vi "Reentrancy Settings for Hierarchy.vi"(8 "error in":errorcluster, 11 "Scratch VI":refnum<vi>) -> (0 "error out":errorcluster, 3 "Reentrancy Settings for VI Hierarchy":T1[](array[typedef]))   [LabVIEW 2009]
uses:
  VI Reentrancy Setting.ctl
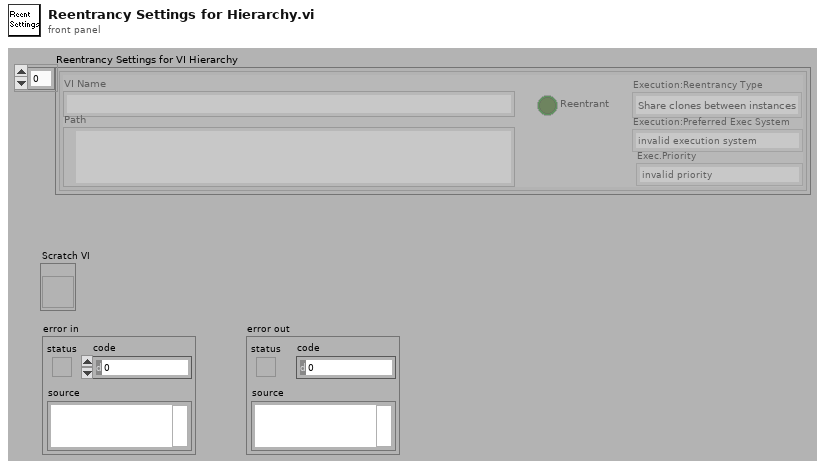
[diagram p1: front panel]
types:
  T1 = typedef "VI Reentrancy Setting.ctl" = cluster{"VI Name":string, "Path":path, "Reentrant":bool, "Execution:Reentrancy Type":enum16{"Share clones between instances", "Preallocate clone for each instance"}, "Execution:Preferred Exec System":enum32{"invalid execution system", "user interface", "standard", "instrument i/o", "data acquisition", "other 1", "other 2", "same as caller"}, "Exec.Priority":enum32{"invalid priority", "background priority", "normal priority", "above normal priority", "high priority", "time critical priority", "subroutine"}}
  T2 = enum8{"Only include commented out diagrams if diagram already loaded", "Never include commented out diagrams", "Always include commented out diagrams"}
  T3 = enum8{"No dynamic dispatch VIs", "Include nearest implementation", "Include all overrides"}
  T4 = enum8{"Include the clone VI", "Include the original reentrant VI instead of the clone VI", "Include both the original reentrant VI and the clone VI"}
  T5 = enum16{"Share clones between instances", "Preallocate clone for each instance"}
  T6 = enum32{"invalid execution system", "user interface", "standard", "instrument i/o", "data acquisition", "other 1", "other 2", "same as caller"}
  T7 = enum32{"invalid priority", "background priority", "normal priority", "above normal priority", "high priority", "time critical priority", "subroutine"}
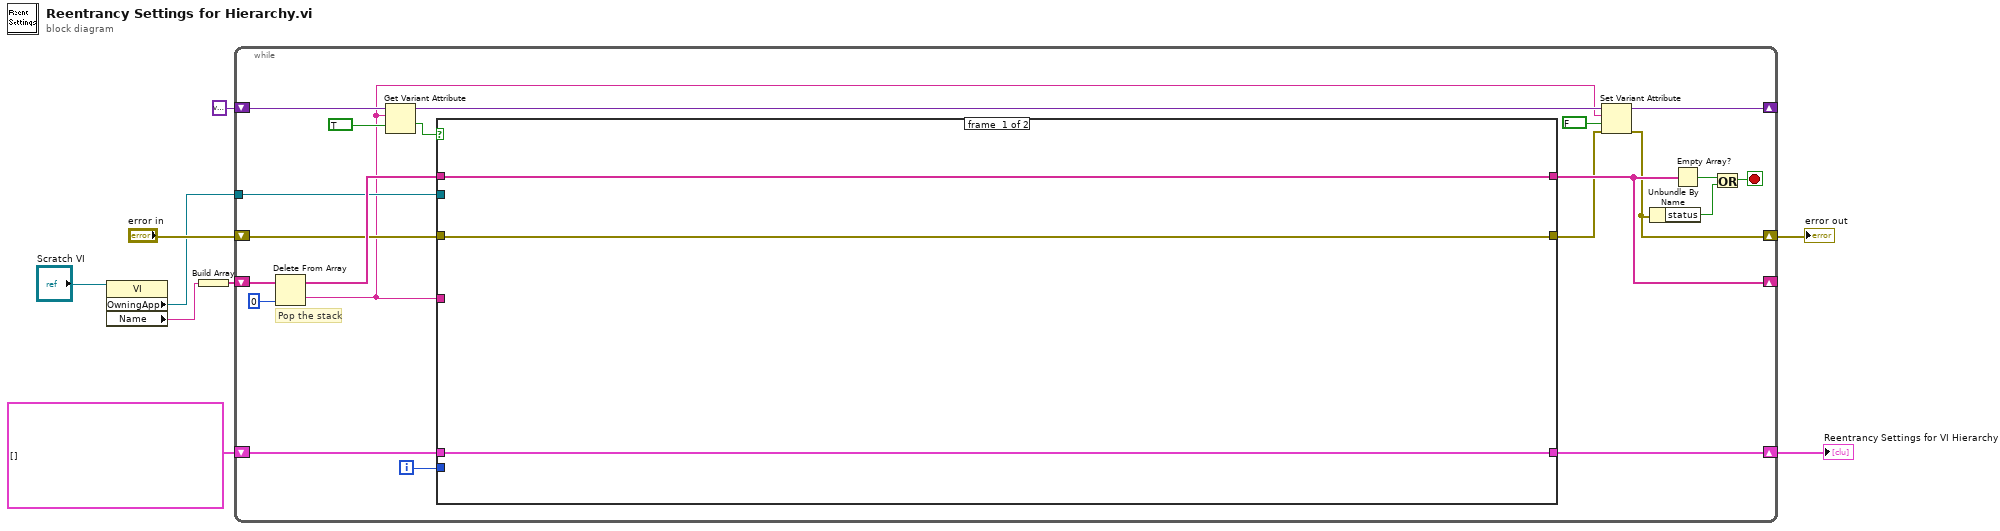
[diagram p0: block diagram]
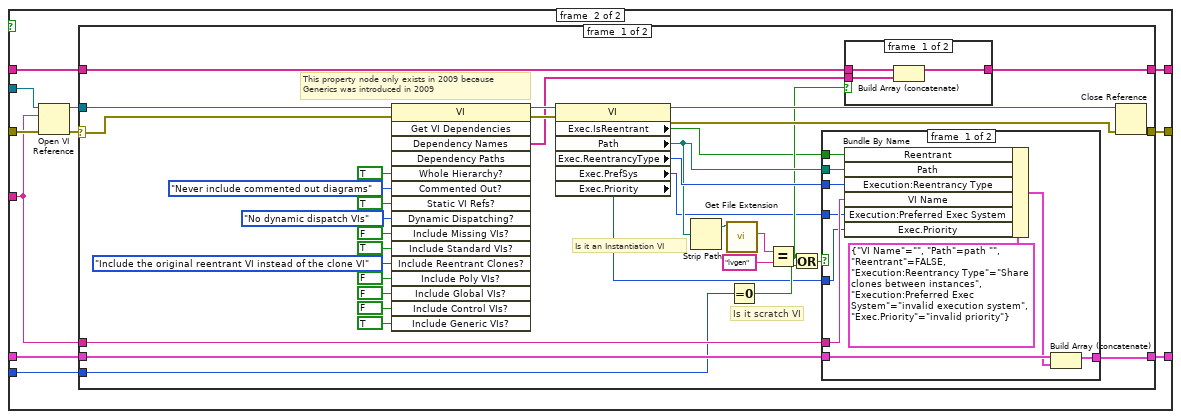
[diagram p2: hidden frame]
diagram:
  n1 = property class="VI"(reference="Scratch VI") -> ("OwningApp"=w2:refnum<vi>, "Name"=w3:string)  [unwired: 1 in, 2 out]
  n2 = Build Array(w3) -> (w4:string[])
  n3 = while {
    shift-right: [w28] -> _
    shift-left: w4 -> [w26]
    shift-right: [w23] -> w9
    shift-left: T1[] [] ("Array") -> [w30]
    shift-right: [w12] -> w8
    shift-left: "error in" -> [w17]
    tunnel: w2 -> [w24]
    shift-right: [w14] -> _
    shift-left: variant -> [w22]
    i -> [w15]
    stop <- w16 stop-if-true
    # "Pop the stack"
    n4 = Delete From Array(array=w26, index=0) -> (deleted portion=w11:string, array with subset deleted=w25:string[])  [unwired: 1 in]
    n5 = Get Variant Attribute(Variant=w22, name=w11, default value (empty Variant)=TRUE) -> (duplicate Variant=w21:variant, value=w19:bool)  [unwired: 1 in, 2 out]
    n6 = case shown="True" w19 {
      tunnel: w30 -> [w31 w36]
      tunnel: [w32 w43] -> w28
      tunnel: [w33 w42] -> w13
      tunnel: w17 -> [w33 w40]
      tunnel: w25 -> [w32 w39]
      tunnel: w24 -> [_ w38]
      tunnel: w11 -> [_ w37]
      tunnel: [w31 w35] -> w23
      tunnel: w15 -> [_ w34]
      frame #0 {
      }
      frame #1 {
        n7 = Open VI Reference(application reference (local)=w38, vi path=w37, error in (no error)=w40) -> (vi reference=w44:refnum<vi>, error out=w41:errorcluster)  [unwired: 3 in]
        n8 = case shown="No Error" w41 {
          selector: w41 -> [w60 w96]
          tunnel: w44 -> [w61 _]
          tunnel: w39 -> [w80 w98]
          tunnel: [w79 w98] -> w43
          tunnel: [w78 w96] -> w42
          tunnel: w37 -> [w77 _]
          tunnel: w36 -> [w76 w97]
          tunnel: [w75 w97] -> w35
          tunnel: w34 -> [w55 _]
          frame #0 {
            # "Is it an Instantiation VI"
            # "Is it scratch VI"
            # "This property node only exists in 2009 because\nGenerics was introduced in 2009"
            n9 = invoke class="VI" method="Get VI Dependencies"(reference=w61, error in=w60, "Whole Hierarchy?"=TRUE, "Commented Out?"=T2."Never include commented out diagrams" ("Commented Out Diagrams?"), "Static VI Refs?"=TRUE, "Dynamic Dispatching?"=T3."No dynamic dispatch VIs", "Include Missing VIs?"=FALSE ("Include Missing Items?"), "Include Standard VIs?"=TRUE, "Include Reentrant Clones?"=T4."Include the original reentrant VI instead of the clone VI", "Include Poly VIs?"=FALSE, "Include Global VIs?"=FALSE, "Include Control VIs?"=FALSE, "Include Generic VIs?"=TRUE) -> (reference out=w58:refnum<vi>, error out=w59:errorcluster, "Dependency Names"=w57:string[])  [unwired: 3 in, 13 out]
            n10 = property class="VI"(reference=w58, error in=w59) -> (reference out=w74:refnum<vi>, error out=w56:errorcluster, "Exec.IsReentrant"=w47:bool, "Path"=w54:path, "Exec.ReentrancyType"=w73:T5, "Exec.PrefSys"=w46:T6, "Exec.Priority"=w45:T7)
            n11 = Strip Path(path=w54) -> (stripped path=w53:path)  [unwired: 1 out]
            n12 = call <vilib>:"Get File Extension.vi"("file"=w53) -> ("lowercase file extension"=w52:string)  [unwired: 7 in, 3 out]
            n13 = Equal To 0?(x=w55) -> (x = 0?=w50:bool)
            n14 = Equal?(x=w52, y="lvgen") -> (x = y?=w48:bool)
            n15 = Or(x=w48, y=w50) -> (x .or. y?=w49:bool)
            n16 = case shown="False" w49 {
              tunnel: w77 -> [w94 _]
              tunnel: w76 -> [w93 w95]
              tunnel: [w92 w95] -> w75
              tunnel: w47 -> [w90 _]
              tunnel: w73 -> [w89 _]
              tunnel: w54 -> [w87 _]
              tunnel: w46 -> [w86 _]
              tunnel: w45 -> [w85 _]
              frame #0 {
                n17 = Bundle By Name(cluster=T1 {"VI Name"="", "Path"=path "", "Reentrant"=FALSE, "Execution:Reentrancy Type"=enum."Share clones between instances", "Execution:Preferred Exec System"=enum."invalid execution system", "Exec.Priority"=enum."invalid priority"}, "Reentrant"=w90, "Path"=w87, "Execution:Reentrancy Type"=w89, "VI Name"=w94, "Execution:Preferred Exec System"=w86, "Exec.Priority"=w85) -> (w91:T1)
                n18 = Build Array (concatenate)(w93, w91) -> (w92:T1[])
              }
              frame #1 {
                # "Do not add InstantiationVIs or\nthe top-level 'scratch' VI to this list"
              }
            }
            n19 = case shown="False" w48 {
              tunnel: w80 -> [w83 w84]
              tunnel: [w82 w84] -> w79
              tunnel: w57 -> [w81 _]
              frame #0 {
                n20 = Build Array (concatenate)(w83, w81) -> (w82:string[])
              }
              frame #1 {
                # "Don't add dependencies\nof Instantiation VIs"
              }
            }
            n21 = Close Reference(reference=w74, error in (no error)=w56) -> (error out=w78:errorcluster)
          }
          frame #1 {
          }
        }
      }
    }
    n22 = Set Variant Attribute(Variant=w21, name=w11, value=FALSE, error in=w13) -> (Variant out=w14:variant, error out=w12:errorcluster)  [unwired: 1 out]
    n23 = Unbundle By Name(w12) -> ("status"=w27:bool)
    n24 = Empty Array?(array=w28) -> (empty?=w29:bool)
    n25 = Or(x=w29, y=w27) -> (x .or. y?=w16:bool)
  }
  "Reentrancy Settings for VI Hierarchy" <- w9
  "error out" <- w8
